vi "Find Page Properties.vi"(8 "error in":errorcluster, 11 "XML File Path":path) -> (0 "error out":errorcluster, 3 "Pages Properties":T1[](array[typedef]))   [LabVIEW 2026, in "NIVS_CDEW_MetaDataObj.lvclass"]
uses:
  NIVS_CDEW_MetaDataObj.lvclass
  Types/Page Properties.ctl
  Types/Page Types.ctl
  Shared/Types/NodeFilteringOptions.ctl
  <vilib>/xml/Load XML File.vi
  <vilib>/xml/Get Node Text Content (String).vi
  NIVS_CDEW_MetaDataObj.lvclass/NIVS_CDEW_MetaDataObj.ctl
  <vilib>/xml/NI_XML.lvlib
  <resource>/objmgr/DOMUserDefRef.rc
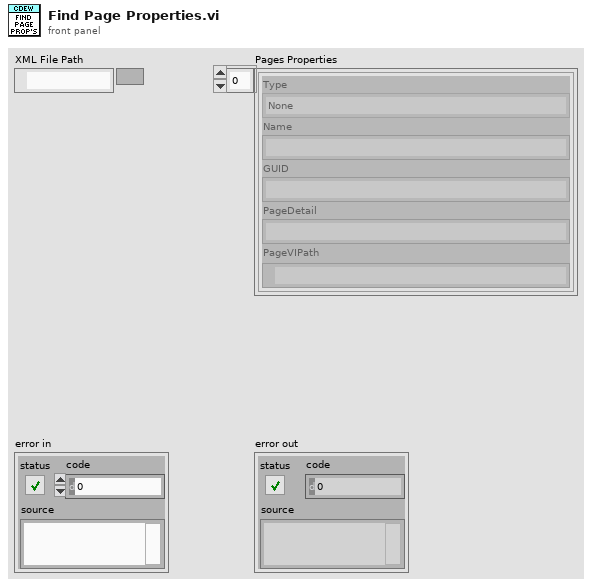
[diagram p1: front panel]
types:
  T1 = typedef "NIVS_CDEW_MetaDataObj.lvclass/Page Properties.ctl" = cluster{"Type":T2, "Name":string, "GUID":string, "PageDetail":string, "PageVIPath":path}
  T2 = typedef "NIVS_CDEW_MetaDataObj.lvclass/Page Types.ctl" = enum16{"None", "CustomDevice", "Channel", "Waveform", "Section", "DynamicChannel", "DynamicWaveform", "DynamicSection"}
  T3 = typedef "NodeFilteringOptions.ctl" = enum16{"GetCustomDeviceNode", "GetAllChannelNodes", "GetAllSectionNodes", "GetAllWaveformNodes", "GetFirstChannelNode", "GetFirstSectionNode", "GetFirstWaveformNode", "GetSpecificSectionNode", "GetSpecificCustomDeviceNode", "GetSpecificChannelNode", "GetSpecificWaveformNode", "GetMatchedNamedNode", "GetEnumDefinitionsNode", "GetSpecificEnumDefinitionNode", "GetAllEnumDefinitionNodes", "GetDynamicChannelNodes"}
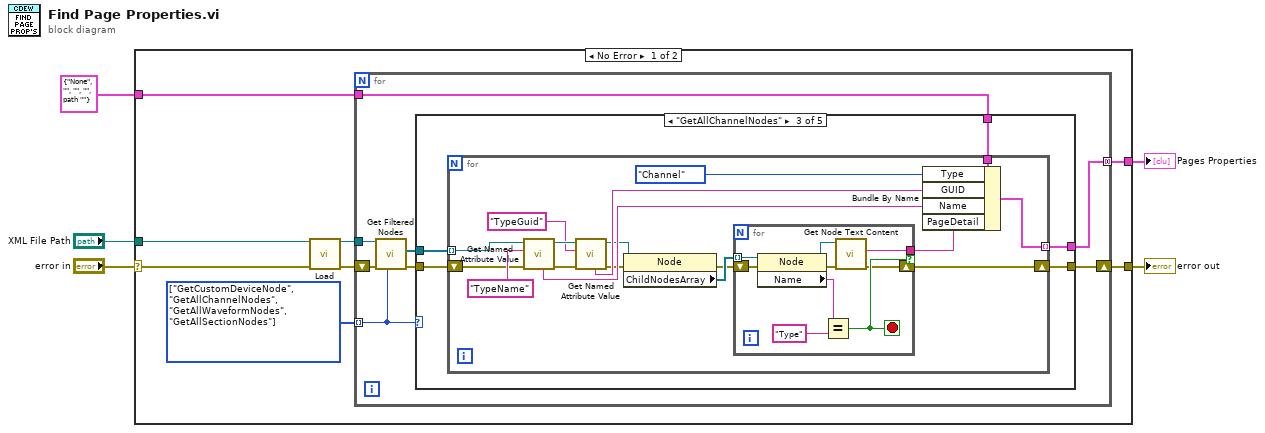
[diagram p0: block diagram]
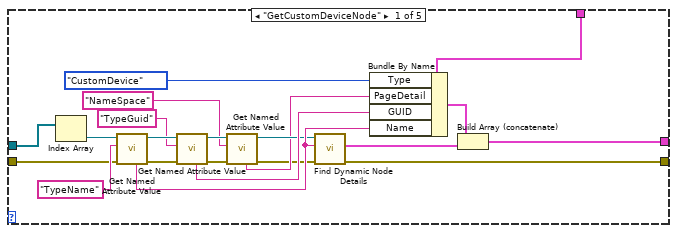
[diagram p2: hidden frame]
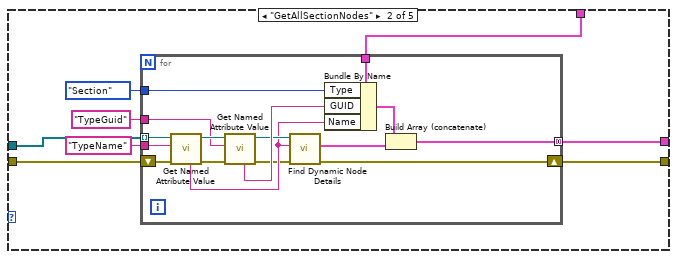
[diagram p3: hidden frame]
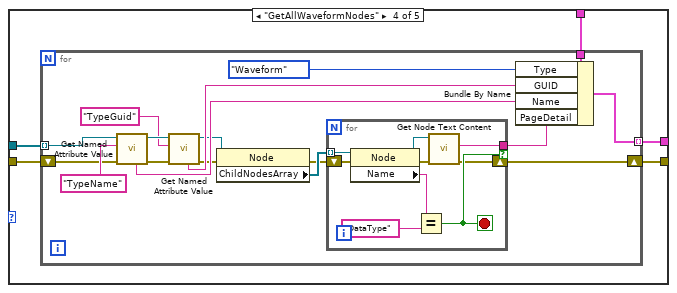
[diagram p4: hidden frame]
diagram:
  n1 = case shown="No Error" "error in" {
    selector: "error in" -> [w7 w130]
    tunnel: "XML File Path" -> [w13 _]
    tunnel: T1 {"Type"=enum."None", "Name"="", "GUID"="", "PageDetail"="", "PageVIPath"=path ""} ("Page Properties") -> [w9 _]
    tunnel: [w8 _] -> w2
    tunnel: [w6 w130] -> w1
    frame No Error {
      w10 = T3[] [enum."GetCustomDeviceNode", enum."GetAllChannelNodes", enum."GetAllWaveformNodes", enum."GetAllSectionNodes"] items=["GetCustomDeviceNode", "GetAllChannelNodes", "GetAllSectionNodes", "GetAllWaveformNodes", "GetFirstChannelNode", "GetFirstSectionNode", "GetFirstWaveformNode", "GetSpecificSectionNode", "GetSpecificCustomDeviceNode", "GetSpecificChannelNode", "GetSpecificWaveformNode", "GetMatchedNamedNode", "GetEnumDefinitionsNode", "GetSpecificEnumDefinitionNode", "GetAllEnumDefinitionNodes", "GetDynamicChannelNodes"]
      n2 = call-poly <vilib>:"Load.vi"("path to XML document"=w13, "error in (no error)"=w7) -> ("DOM document out"=w12:refnum<k20>, "error out"=w11:errorcluster)  [unwired: 11 in, 1 out]
      n3 = for {
        tunnel: w12 -> [w21]
        tunnel: w10 -> [w18] mode=indexing
        tunnel: w9 -> [w17]
        tunnel: [w16] -> w8 mode=concatenating
        shift-right: [w14] -> w6
        shift-left: w11 -> [w20]
        n4 = call "Get Filtered Nodes.vi"("Node Filtering"=w18, "error in"=w20, "Document in"=w21) -> ("error out"=w15:errorcluster, "Filtered Nodes"=w19:refnum<k20>[])  [unwired: 4 in, 3 out]
        n5 = case shown="\"GetAllChannelNodes\"" w18 {
          tunnel: w19 -> [w42 w50 w71 w102 _]
          tunnel: w17 -> [w41 w48 w69 w100 _]
          tunnel: [w35 w49 w70 w101 _] -> w16
          tunnel: w15 -> [w26 w44 w68 w99 w129]
          tunnel: [w22 w43 w67 w98 w129] -> w14
          frame "GetCustomDeviceNode" {
            n6 = Index Array(array=w42) -> (element=w33:refnum<k20>)  [unwired: 1 in]
            n7 = call "Get Named Attribute Value.vi"("error in"=w26, "Attribute Name"="TypeName", "Node In"=w33) -> ("error out"=w25:errorcluster, "Node Out"=w38:refnum<k20>, "Attribute Value"=w31:string)  [unwired: 5 in, 1 out]
            n8 = call "Get Named Attribute Value.vi"("error in"=w25, "Attribute Name"="TypeGuid", "Node In"=w38) -> ("error out"=w24:errorcluster, "Node Out"=w30:refnum<k20>, "Attribute Value"=w39:string)  [unwired: 5 in, 1 out]
            n9 = call "Get Named Attribute Value.vi"("error in"=w24, "Attribute Name"="NameSpace", "Node In"=w30) -> ("error out"=w23:errorcluster, "Node Out"=w29:refnum<k20>, "Attribute Value"=w27:string)  [unwired: 5 in, 1 out]
            n10 = call "Find Dynamic Node Details.vi"("error in"=w23, "Parent Node"=w31, "Node In"=w29) -> ("error out"=w22:errorcluster, "Dynamic Page Properties"=w32:T1[])  [unwired: 7 in]
            n11 = Bundle By Name(cluster=w41, "Type"=Page_Types."CustomDevice", "PageDetail"=w27, "GUID"=w39, "Name"=w31) -> (w36:T1)
            n12 = Build Array (concatenate)(w36, w32) -> (w35:T1[])
          }
          frame "GetAllSectionNodes" {
            n13 = for {
              tunnel: w50 -> [w64] mode=indexing
              tunnel: [w55] -> w49 mode=concatenating
              tunnel: w48 -> [w63]
              tunnel: "TypeName" ("Attribute Name") -> [w62]
              tunnel: "TypeGuid" ("Attribute Name") -> [w61]
              tunnel: Page_Types."Section" ("Type") -> [w60]
              shift-right: [w51] -> w43
              shift-left: w44 -> [w54]
              n14 = call "Get Named Attribute Value.vi"("error in"=w54, "Attribute Name"=w62, "Node In"=w64) -> ("error out"=w53:errorcluster, "Node Out"=w65:refnum<k20>, "Attribute Value"=w58:string)  [unwired: 5 in, 1 out]
              n15 = call "Get Named Attribute Value.vi"("error in"=w53, "Attribute Name"=w61, "Node In"=w65) -> ("error out"=w52:errorcluster, "Node Out"=w59:refnum<k20>, "Attribute Value"=w66:string)  [unwired: 5 in, 1 out]
              n16 = call "Find Dynamic Node Details.vi"("error in"=w52, "Parent Node"=w58, "Node In"=w59) -> ("error out"=w51:errorcluster, "Dynamic Page Properties"=w57:T1[])  [unwired: 7 in]
              n17 = Bundle By Name(cluster=w63, "Type"=w60, "GUID"=w66, "Name"=w58) -> (w56:T1)
              n18 = Build Array (concatenate)(w56, w57) -> (w55:T1[])
            }
          }
          frame "GetAllChannelNodes" {
            n19 = for {
              tunnel: w71 -> [w82] mode=indexing
              tunnel: [w81] -> w70 mode=indexing
              tunnel: w69 -> [w80]
              shift-right: [w72] -> w67
              shift-left: w68 -> [w76]
              n20 = call "Get Named Attribute Value.vi"("error in"=w76, "Attribute Name"="TypeName", "Node In"=w82) -> ("error out"=w75:errorcluster, "Node Out"=w84:refnum<k20>, "Attribute Value"=w87:string)  [unwired: 5 in, 1 out]
              n21 = call "Get Named Attribute Value.vi"("error in"=w75, "Attribute Name"="TypeGuid", "Node In"=w84) -> ("error out"=w74:errorcluster, "Node Out"=w79:refnum<k20>, "Attribute Value"=w86:string)  [unwired: 5 in, 1 out]
              n22 = property class="Node"(reference=w79, error in=w74) -> (error out=w73:errorcluster, "ChildNodesArray"=w78:refnum<k20>[])  [unwired: 1 out]
              n23 = for {
                tunnel: w78 -> [w97] mode=indexing
                tunnel: [w92] -> w77 if=w94
                shift-right: [w91] -> w72
                shift-left: w73 -> [w90]
                stop <- w94 stop-if-true
                n24 = property class="Node"(reference=w97, error in=w90) -> (reference out=w93:refnum<k20>, error out=w89:errorcluster, "Name"=w96:string)
                n25 = Equal?(x=w96, y="Type") -> (x = y?=w94:bool)
                n26 = call-poly <vilib>:"Get Node Text Content.vi"("error in (no error)"=w89, "node in"=w93) -> ("error out"=w91:errorcluster, "node text"=w92:string)  [unwired: 7 in, 1 out]
              }
              n27 = Bundle By Name(cluster=w80, "Type"=Page_Types."Channel", "GUID"=w86, "Name"=w87, "PageDetail"=w77) -> (w81:T1)
            }
          }
          frame "GetAllWaveformNodes" {
            n28 = for {
              tunnel: w102 -> [w113] mode=indexing
              tunnel: [w112] -> w101 mode=indexing
              tunnel: w100 -> [w111]
              shift-right: [w103] -> w98
              shift-left: w99 -> [w107]
              n29 = call "Get Named Attribute Value.vi"("error in"=w107, "Attribute Name"="TypeName", "Node In"=w113) -> ("error out"=w106:errorcluster, "Node Out"=w115:refnum<k20>, "Attribute Value"=w118:string)  [unwired: 5 in, 1 out]
              n30 = call "Get Named Attribute Value.vi"("error in"=w106, "Attribute Name"="TypeGuid", "Node In"=w115) -> ("error out"=w105:errorcluster, "Node Out"=w110:refnum<k20>, "Attribute Value"=w117:string)  [unwired: 5 in, 1 out]
              n31 = property class="Node"(reference=w110, error in=w105) -> (error out=w104:errorcluster, "ChildNodesArray"=w109:refnum<k20>[])  [unwired: 1 out]
              n32 = for {
                tunnel: w109 -> [w128] mode=indexing
                tunnel: [w123] -> w108 if=w125
                shift-right: [w122] -> w103
                shift-left: w104 -> [w121]
                stop <- w125 stop-if-true
                n33 = property class="Node"(reference=w128, error in=w121) -> (reference out=w124:refnum<k20>, error out=w120:errorcluster, "Name"=w127:string)
                n34 = Equal?(x=w127, y="DataType") -> (x = y?=w125:bool)
                n35 = call-poly <vilib>:"Get Node Text Content.vi"("error in (no error)"=w120, "node in"=w124) -> ("error out"=w122:errorcluster, "node text"=w123:string)  [unwired: 7 in, 1 out]
              }
              n36 = Bundle By Name(cluster=w111, "Type"=Page_Types."Waveform", "GUID"=w117, "Name"=w118, "PageDetail"=w108) -> (w112:T1)
            }
          }
          frame Default {
          }
        }
      }
    }
    frame Error {
    }
  }
  "Pages Properties" <- w2
  "error out" <- w1
